vi "MGI Get VI Control Ref[].vi"(8 "error in":errorcluster, 9 "Include Tab Page Controls? (T)":bool=TRUE, 11 "VI (Caller)":refnum<vi>) -> (0 "error out":errorcluster, 1 "Control Type[i]":T1[](array[typedef]), 2 "Control Label Chain[i]":string[](array[string]), 3 "Control[i]":refnum<vi>[](array[refnum]))   [LabVIEW 2016]
doc: "Returns refnums of all controls on a front panel. If <B>Include Tab Page Controls</B> is true, then all controls on tab pages are included recursively.\nThe type of each returned refnum is also output in <B>Control Type[i]</B>. <B>Control Label[i]</B> contains the label of each control.\n\nAuthored by Martin Weiss, Shawn Walpole\nsupport@mooregoodideas.com\nwww.mooregoodideas.com\n\nCopyright (c) 2010, Moore Good Ideas, Inc.\n\nAll rights reserved.\n\nRedistribution and use in source and binary forms, with or without modification, are permitted provided that the following conditions are met:\n\n * Redistributions of source code must retain the above copyright notice, this list of conditions and the following disclaimer.\n * Redistributions in binary form must reproduce the above copyright notice, this list of conditions and the following disclaimer in the documentation and/or other materials provided with the distribution.\n * Neither the name of Moore Good Ideas, Inc. nor the names of its contributors may be used to endorse or promote products derived from this software without specific prior written permission.\n\nTHIS SOFTWARE IS PROVIDED BY THE COPYRIGHT HOLDERS AND CONTRIBUTORS \"AS IS\" AND ANY EXPRESS OR IMPLIED WARRANTIES, INCLUDING, BUT NOT LIMITED TO, THE IMPLIED WARRANTIES OF MERCHANTABILITY AND FITNESS FOR A PARTICULAR PURPOSE ARE DISCLAIMED. IN NO EVENT SHALL THE COPYRIGHT OWNER OR CONTRIBUTORS BE LIABLE FOR ANY DIRECT, INDIRECT, INCIDENTAL, SPECIAL, EXEMPLARY, OR CONSEQUENTIAL DAMAGES (INCLUDING, BUT NOT LIMITED TO, PROCUREMENT OF SUBSTITUTE GOODS OR SERVICES; LOSS OF USE, DATA, OR PROFITS; OR BUSINESS INTERRUPTION) HOWEVER CAUSED AND ON ANY THEORY OF LIABILITY, WHETHER IN CONTRACT, STRICT LIABILITY, OR TORT (INCLUDING NEGLIGENCE OR OTHERWISE) ARISING IN ANY WAY OUT OF THE USE OF THIS SOFTWARE, EVEN IF ADVISED OF THE POSSIBILITY OF SUCH DAMAGE."
uses:
  <userlib>/_OpenG.lib/appcontrol/appcontrol.llb/ClassID Names Enum__ogtk.ctl
  <userlib>/_MGI/Application Control/MGI VI Reference/MGI Caller's VI Reference.vi
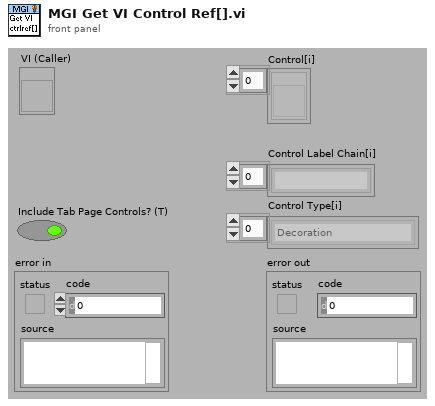
[diagram p1: front panel]
types:
  T1 = typedef "ClassID Names Enum__ogtk.ctl" = enum32{"0 <undefined>", "1 <undefined>", "2 <undefined>", "Generic", "Decoration", "Text", "Control", "ColorBox", "Boolean", "RefNum", "Variant", "Path", "ListBox", "Table", "Array", "Picture", "ActiveXContainer", "Numeric", "Digital", "NamedNumeric", "ColorRamp", "Slide", "GraphOrChart", "WaveformChart", "WaveformGraph", "IntensityChart", "IntensityGraph", "String", "IOName", "ComboBox", "Cluster", "Panel", "Knob", "NumWithScale", "Ring", "Enum", "GObject", "Plot", "Cursor", "NumericText", "Scale", "ColorScale", "GraphScale", "ColorGraphScale", "TypedRefNum", "OldKnobScale", "MCListbox", "MeasureData", "BVTag", "DAQName", "VISAName", "IVIName", "SlideScale", "TabControl", "Page", "TabArrayTabControl", "ConPane"}
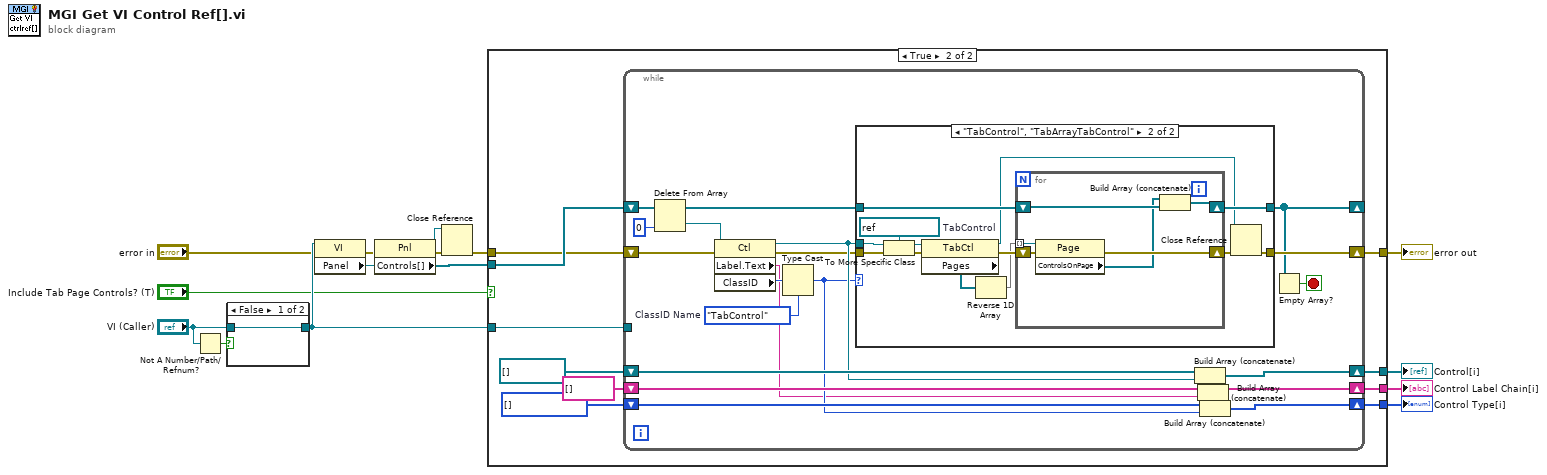
[diagram p0: block diagram]
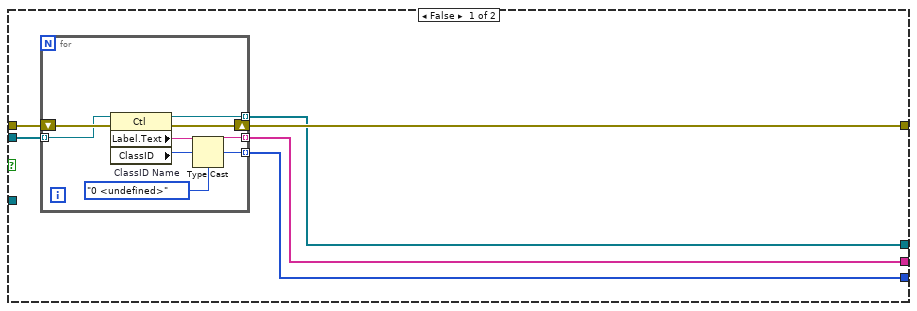
[diagram p2: hidden frame]
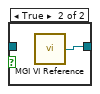
[diagram p4: hidden frame]
diagram:
  n1 = Not A Number/Path/Refnum?(number/path/refnum="VI (Caller)") -> (NaN/Path/Refnum?=w13:bool)
  n2 = case shown="False" w13 {
    tunnel: "VI (Caller)" -> [w16 _]
    tunnel: [w16 w17] -> w9
    frame False {
    }
    frame True {
      n3 = call-poly <userlib>:"MGI VI Reference.vi"() -> ("Caller's VI Reference"=w17:refnum<vi>)  [unwired: 1 in]
    }
  }
  n4 = property class="VI"(reference=w9, error in="error in") -> (error out=w10:errorcluster, "Panel"=w11:refnum<vi>)  [unwired: 1 out]
  n5 = property class="Pnl"(reference=w11, error in=w10) -> (reference out=w5:refnum<vi>, error out=w7:errorcluster, "Controls[]"=w1:refnum<vi>[])
  n6 = Close Reference(reference=w5, error in (no error)=w7) -> (error out=w6:errorcluster)
  n7 = case shown="True" "Include Tab Page Controls? (T)" {
    tunnel: [w21 w41] -> w15
    tunnel: [w20 w36] -> w14
    tunnel: w9 -> [_ w40]
    tunnel: w1 -> [w23 w39]
    tunnel: w6 -> [w22 w38]
    tunnel: [w19 w34] -> w3
    tunnel: [w18 w33] -> w2
    frame False {
      n8 = for {
        tunnel: w23 -> [w24] mode=indexing
        shift-right: [w31] -> w21
        shift-left: w22 -> [w30]
        tunnel: [w29] -> w19 mode=indexing
        tunnel: [w25] -> w18 mode=indexing
        tunnel: [w28] -> w20 mode=indexing
        w27 = ClassID_Names_Enum__ogtk."0 <undefined>"  # ClassID Name
        n9 = property class="Ctl"(reference=w24, error in=w30) -> (reference out=w28:refnum<vi>, error out=w31:errorcluster, "Label.Text"=w29:string, "ClassID"=w26:u32)
        n10 = Type Cast(type=w27, x=w26) -> (*(type *) &x=w25:T1)
      }
    }
    frame True {
      w32 = T1[] [] items=["0 <undefined>", "1 <undefined>", "2 <undefined>", "Generic", "Decoration", "Text", "Control", "ColorBox", "Boolean", "RefNum", "Variant", "Path", "ListBox", "Table", "Array", "Picture", "ActiveXContainer", "Numeric", "Digital", "NamedNumeric", "ColorRamp", "Slide", "GraphOrChart", "WaveformChart", "WaveformGraph", "IntensityChart", "IntensityGraph", "String", "IOName", "ComboBox", "Cluster", "Panel", "Knob", "NumWithScale", "Ring", "Enum", "GObject", "Plot", "Cursor", "NumericText", "Scale", "ColorScale", "GraphScale", "ColorGraphScale", "TypedRefNum", "OldKnobScale", "MCListbox", "MeasureData", "BVTag", "DAQName", "VISAName", "IVIName", "SlideScale", "TabControl", "Page", "TabArrayTabControl", "ConPane"]
      n11 = while {
        tunnel: w40 -> [_]
        shift-right: [w56] -> _
        shift-left: w39 -> [w60]
        shift-right: [w61] -> w41
        shift-left: w38 -> [w46]
        shift-right: [w54] -> w36
        shift-left: refnum<vi>[] [] -> [w57]
        shift-right: [w50] -> w34
        shift-left: string[] [] -> [w49]
        shift-right: [w48] -> w33
        shift-left: w32 -> [w47]
        stop <- w55 stop-if-true
        w51 = ClassID_Names_Enum__ogtk."TabControl"  # ClassID Name
        n12 = Delete From Array(array=w60, index=0) -> (deleted portion=w43:refnum<vi>, array with subset deleted=w58:refnum<vi>[])  [unwired: 1 in]
        n13 = property class="Ctl"(reference=w43, error in=w46) -> (reference out=w53:refnum<vi>, error out=w45:errorcluster, "Label.Text"=w42:string, "ClassID"=w52:u32)
        n14 = Type Cast(type=w51, x=w52) -> (*(type *) &x=w44:T1)
        n15 = case shown="\"TabControl\", \"TabArrayTabControl\"" w44 {
          tunnel: [w62 w76] -> w61
          tunnel: w58 -> [w63 w75]
          tunnel: [w63 w72] -> w56
          tunnel: w53 -> [_ w71]
          tunnel: w45 -> [w62 w66]
          frame Default {
          }
          frame "TabControl", "TabArrayTabControl" {
            w73 = refnum<vi> refnum  # TabControl
            n16 = To More Specific Class(target class=w73, reference=w71, error in=w66) -> (specific class reference=w74:refnum<vi>, error out=w67:errorcluster)
            n17 = property class="TabCtl"(reference=w74, error in=w67) -> (reference out=w69:refnum<vi>, error out=w70:errorcluster, "Pages"=w65:refnum<vi>[])
            n18 = Reverse 1D Array(array=w65) -> (reversed array=w64:refnum<vi>[])
            n19 = for {
              tunnel: w64 -> [w82] mode=indexing
              shift-right: [w80] -> w68
              shift-left: w70 -> [w81]
              shift-right: [w79] -> w72
              shift-left: w75 -> [w78]
              n20 = property class="Page"(reference=w82, error in=w81) -> (error out=w80:errorcluster, "ControlsOnPage"=w77:refnum<vi>[])  [unwired: 1 out]
              n21 = Build Array (concatenate)(w77, w78) -> (w79:refnum<vi>[])
            }
            n22 = Close Reference(reference=w69, error in (no error)=w68) -> (error out=w76:errorcluster)
          }
        }
        n23 = Build Array (concatenate)(w57, w53) -> (w54:refnum<vi>[])
        n24 = Build Array (concatenate)(w49, w42) -> (w50:string[])
        n25 = Build Array (concatenate)(w47, w44) -> (w48:T1[])
        n26 = Empty Array?(array=w56) -> (empty?=w55:bool)
      }
    }
  }
  "error out" <- w15
  "Control[i]" <- w14
  "Control Type[i]" <- w2
  "Control Label Chain[i]" <- w3
